vi "SinCos1.vi"() -> (8 "SinCos1":refnum<class "SinCos1.lvclass">)   [LabVIEW 2017, in "SinCos1.lvclass"]
uses:
  SinCos1.lvclass
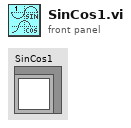
[diagram p1: front panel]
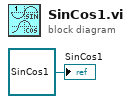
[diagram p0: block diagram]
diagram:
  "SinCos1" <- refnum<class "SinCos1.lvclass"> refnum ("SinCos1.lvclass")
